vi "JSON ParserDTCMap.vi"(8 "Error In":errorcluster, 9 "NumElements":i32=24, 10 "jsonin":string, 11 "Sequence Context In":refnum<k7>) -> (0 "error out":errorcluster, 1 "Status":dbl[](array[numeric]), 2 "Final":u32[](array[numeric]), 3 "Initial":u32[](array[numeric]), 4 "Map_Defs":string[](array[string]), 5 "output cluster":cluster{string[], i32[]})   [LabVIEW 2017]
panel:
  out "Parameter Set":string
  out "output array":string[][](array[string])
  out "Param Values":string[](array[string])
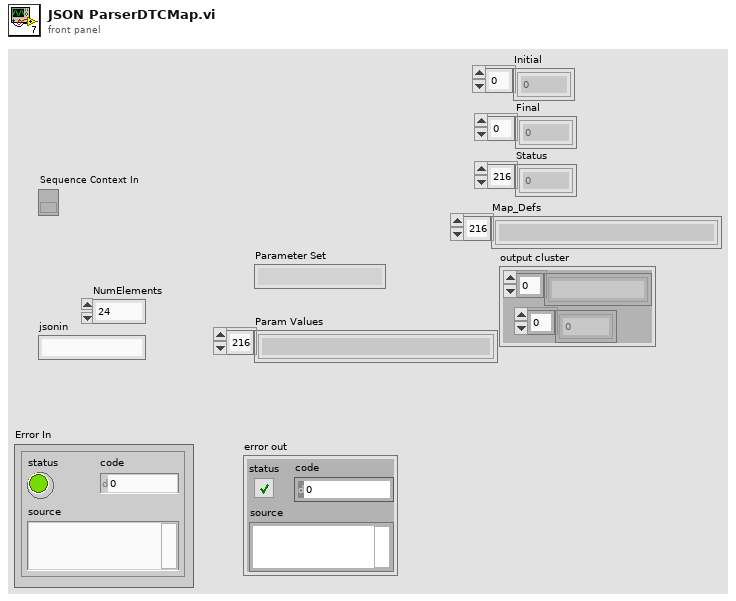
[diagram p1: front panel]
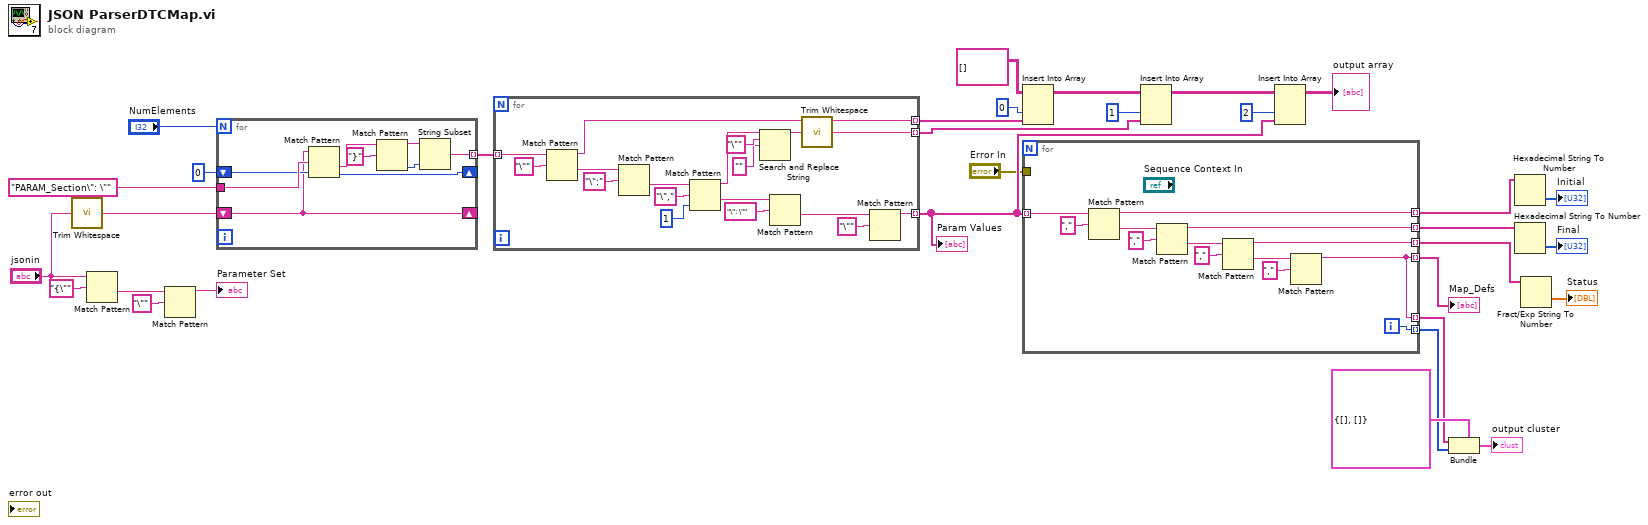
[diagram p0: block diagram]
diagram:
  n1 = call <vilib>:"Trim Whitespace.vi"("string"="jsonin") -> ("trimmed string"=w29:string)  [unwired: 1 in]
  n2 = Match Pattern(string="jsonin", regular expression="{\"") -> (after substring=w17:string)  [unwired: 1 in, 3 out]
  n3 = Match Pattern(string=w17, regular expression="\"") -> (before substring=→"Parameter Set":string)  [unwired: 1 in, 3 out]
  n4 = for {
    N: "NumElements" -> [_]
    tunnel: "PARAM_Section\": \"" ("regular expression") -> [w41]
    shift-right: [w34] -> _
    shift-left: 0 -> [w35]
    tunnel: [w37] -> w30 mode=indexing
    shift-right: [w33] -> _
    shift-left: w29 -> [w33]
    n5 = Match Pattern(string=w33, regular expression=w41, offset (0)=w35) -> (after substring=w40:string, offset past match=w34:i32)  [unwired: 2 out]
    n6 = Match Pattern(string=w40, regular expression="}") -> (before substring=w38:string, offset past match=w36:i32)  [unwired: 1 in, 2 out]
    n7 = String Subset(string=w38, length (rest)=w36) -> (substring=w37:string)  [unwired: 1 in]
  }
  n8 = for {
    tunnel: w30 -> [w46] mode=indexing
    tunnel: [w44] -> w13 mode=indexing
    tunnel: [w43] -> w26 mode=indexing
    tunnel: [w42] -> w23 mode=indexing
    n9 = Match Pattern(string=w46, regular expression="\"") -> (before substring=w43:string, after substring=w58:string)  [unwired: 1 in, 2 out]
    n10 = Match Pattern(string=w58, regular expression="\":") -> (after substring=w56:string)  [unwired: 1 in, 3 out]
    n11 = Match Pattern(string=w56, regular expression="\",", offset (0)=1) -> (before substring=w53:string, after substring=w49:string)  [unwired: 2 out]
    n12 = Search and Replace String(input string=w53, search string="\"", replace string="" ("replace string (\"\")")) -> (result string=w50:string)  [unwired: 5 in, 3 out]
    n13 = Match Pattern(string=w49, regular expression="\": \"") -> (after substring=w45:string)  [unwired: 1 in, 3 out]
    n14 = call <vilib>:"Trim Whitespace.vi"("string"=w50) -> ("trimmed string"=w42:string)  [unwired: 1 in]
    n15 = Match Pattern(string=w45, regular expression="\"") -> (before substring=w44:string)  [unwired: 1 in, 3 out]
  }
  "Param Values" <- w13
  n16 = Insert Into Array(array=string[][] [], index (col)=0 ("disabled index (col)"), new element=w26) -> (w24:string[][])  [unwired: 1 in]
  n17 = for {
    tunnel: w13 -> [w72] mode=indexing
    tunnel: [w61] -> w12 mode=indexing
    tunnel: [w64] -> w11 mode=indexing
    tunnel: [w63] -> w9 mode=indexing
    tunnel: [w62] -> w2 mode=indexing
    tunnel: "Error In" -> [_]
    tunnel: [w61] -> w5 mode=indexing
    tunnel: [w60] -> w4 mode=indexing
    i -> [w60]
    n18 = Match Pattern(string=w72, regular expression=",") -> (before substring=w64:string, after substring=w69:string)  [unwired: 1 in, 2 out]
    n19 = Match Pattern(string=w69, regular expression=",") -> (before substring=w63:string, after substring=w68:string)  [unwired: 1 in, 2 out]
    n20 = Match Pattern(string=w68, regular expression=",") -> (before substring=w62:string, after substring=w66:string)  [unwired: 1 in, 2 out]
    n21 = Match Pattern(string=w66, regular expression=",") -> (before substring=w61:string)  [unwired: 1 in, 3 out]
  }
  "Map_Defs" <- w12
  n22 = Insert Into Array(array=w24, index (col)=1 ("disabled index (col)"), new element=w23) -> (w21:string[][])  [unwired: 1 in]
  n23 = Insert Into Array(array=w21, index (col)=2 ("disabled index (col)"), new element=w13) -> (→"output array":string[][])  [unwired: 1 in]
  n24 = Bundle(cluster=cluster{string[], i32[]} {[], []}, w5, w4) -> (→"output cluster":cluster{string[], i32[]})
  n25 = Hexadecimal String To Number(string=w11) -> (number=→"Initial":u32[])  [unwired: 2 in, 1 out]
  n26 = Hexadecimal String To Number(string=w9) -> (number=→"Final":u32[])  [unwired: 2 in, 1 out]
  n27 = Fract/Exp String To Number(string=w2) -> (number=→"Status":dbl[])  [unwired: 3 in, 1 out]
